vi "Scan Engine Custom IO - To FPGA.vi"(8 "error in (no error)":errorcluster, 11 "Node Ptr":T1 format="%.0x") -> (0 "error out":errorcluster)   [LabVIEW 2016, in "Scan Engine Custom Device.lvlib"]
uses:
  Scan Engine Custom Device.lvlib
  <vilib>/NI Veristand/Custom Device API/Custom Device Item Ref.ctl
  Type Defs/UDV Data Type.ctl
  Type Defs/FXP Config.ctl
  Globals/Property Strings.vi
  <vilib>/NI Veristand/Custom Device API/Get Item Property (String).vi
  <vilib>/NI Veristand/Custom Device API/Get Item Property (U16).vi
  <vilib>/NI Veristand/Custom Device API/Get Item Property (Variant).vi
  <vilib>/NI Veristand/Custom Device API/Custom Device API.lvlib
panel:
  out "IO Variable Name":string
  in  "Default Value":dbl
  in  "Units":string
  out "Data Type":string
  in  "Header":cluster{"Section Name":string}={"Section Name"="Custom FPGA I/O"}
  in  "Description":string
  in  "Name":string
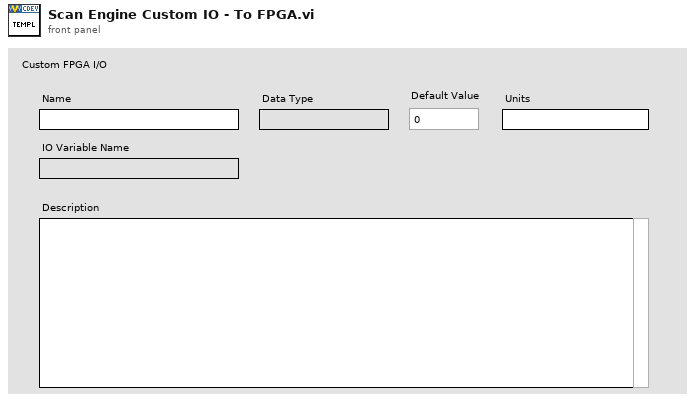
[diagram p1: front panel]
types:
  T1 = typedef "Custom Device API.lvlib/Custom Device Item Ref.ctl" = u64
  T2 = typedef "Scan Engine Custom Device.lvlib/UDV Data Type.ctl" = enum16{"Boolean", "Fixed Point", "Int8", "Int16", "Int32", "Int64", "U32 Bit Field", "UInt8", "UInt16", "UInt32", "UInt64", "Other"}
  T3 = typedef "Custom Device API.lvlib/Custom Device Item Info.ctl" = cluster{"Name":string, "Is Channel":bool, "GUID":string, "Is Waveform":bool}
  T4 = typedef "Custom Device API.lvlib/Custom Device Channel.ctl" = cluster{"Type":T5, "Units":string, "Default Value":dbl, "Faultable":bool, "Scalable":bool}
  T5 = typedef "Custom Device API.lvlib/Custom Device Channel Type.ctl" = enum16{"Input", "Output"}
  T6 = typedef "Scan Engine Custom Device.lvlib/FXP Config.ctl" = cluster{"signed":bool, "size":u32, "integersize":i32}
  T7 = typedef "Custom Device API.lvlib/Custom Device Commands.ctl" = enum16{"Default", "Item renamed", "Shutdown", "Dynamic button pressed"}
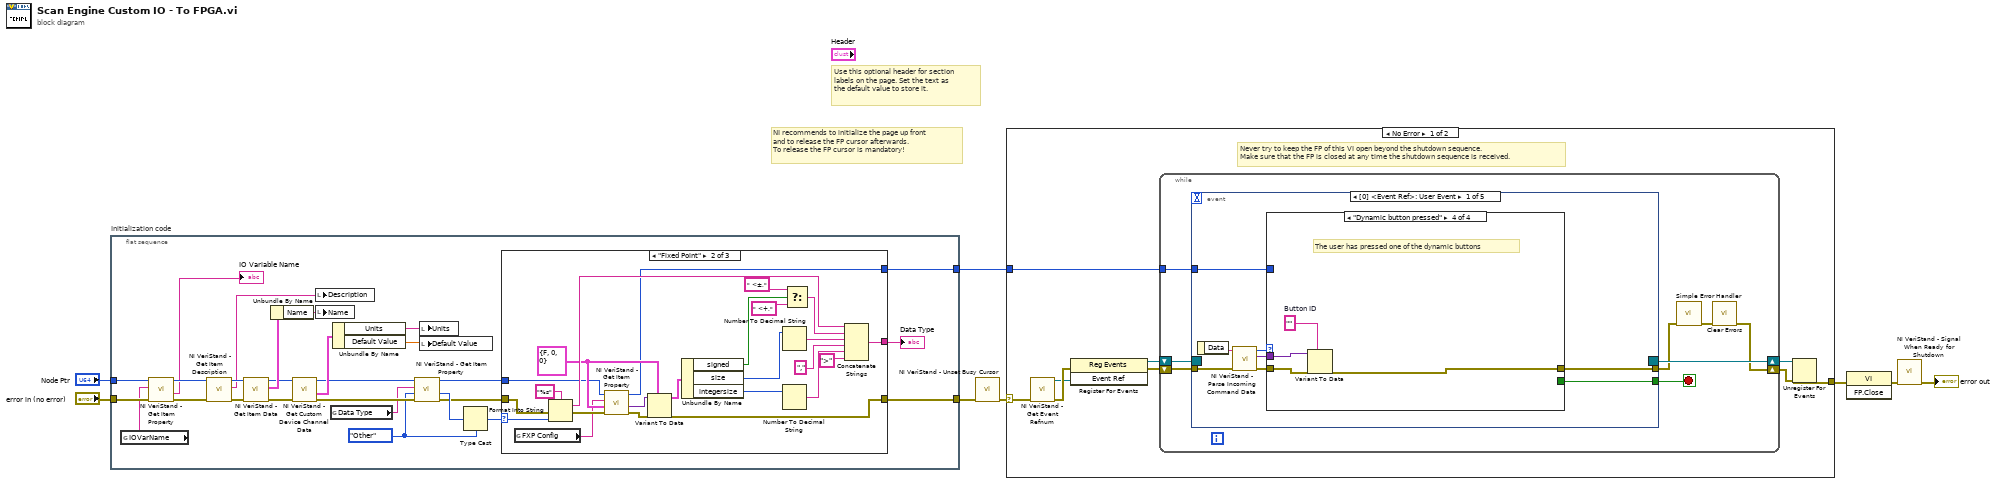
[diagram p0: block diagram]
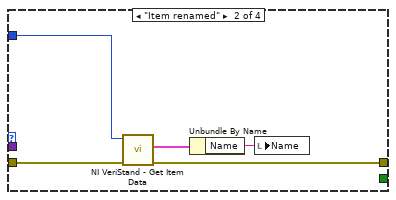
[diagram p3: hidden frame]
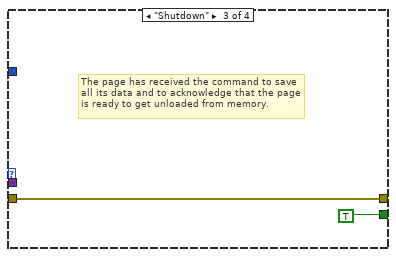
[diagram p4: hidden frame]
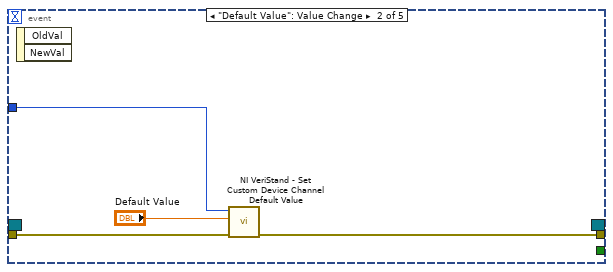
[diagram p5: hidden frame]
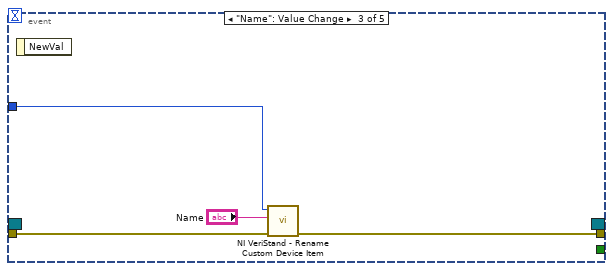
[diagram p6: hidden frame]
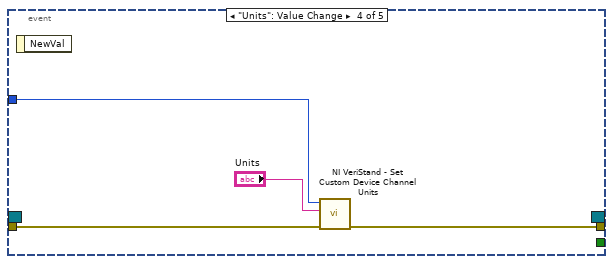
[diagram p7: hidden frame]
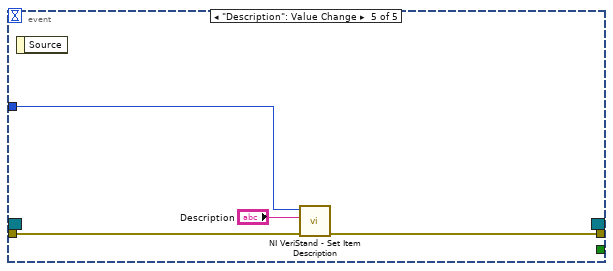
[diagram p8: hidden frame]
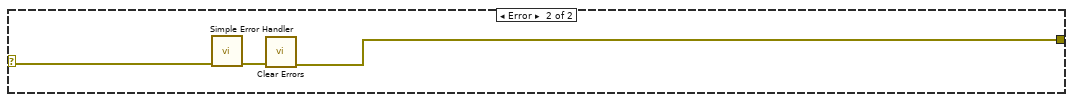
[diagram p9: hidden frame]
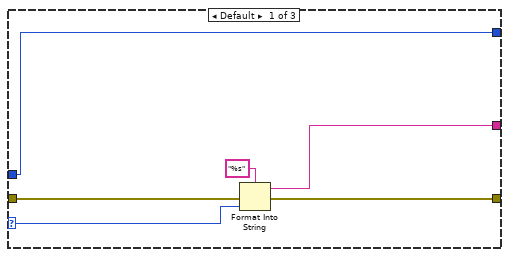
[diagram p10: hidden frame]
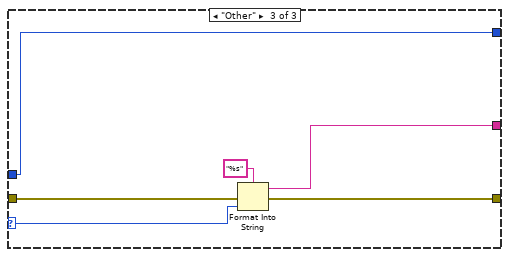
[diagram p11: hidden frame]
diagram:
  # "Use this optional header for section labels on the page. Set the text as the default value to store it."
  # "NI recommends to initialize the page up front\nand to release the FP cursor afterwards.\nTo release the FP cursor is mandatory!"
  n1 = flat-sequence "Initialization code" {
    tunnel: "error in (no error)" -> [w14]
    tunnel: "Node Ptr" -> [w12]
    tunnel: [w18] -> w4
    tunnel: [w16] -> w1
    frame #0 {
      w22 = UDV_Data_Type."Other" ("UDV Data Type out")
      n2 = global read "Property Strings.vi" "IOVarName"() -> (w9:string)
      n3 = call-poly <vilib>:"NI VeriStand - Get Item Property.vi"("error in (no error)"=w14, "Property Name"=w9, "Item Ref in"=w12) -> ("error out"=w13:errorcluster, "Value"=→"IO Variable Name":string, "Item Ref out"=w11:T1)  [unwired: 5 in, 1 out]
      n4 = call <vilib>:"NI VeriStand - Get Item Description.vi"("error in (no error)"=w13, "Item Ref in"=w11) -> ("error out"=w33:errorcluster, "Description"=w34:string, "Item Ref out"=w35:T1)  [unwired: 7 out]
      n5 = call <vilib>:"NI VeriStand - Get Item Data.vi"("error in (no error)"=w33, "Item Ref in"=w35) -> ("error out"=w29:errorcluster, "Item Info"=w32:T3, "Item Ref out"=w30:T1)  [unwired: 7 out]
      n6 = Unbundle By Name(w32) -> ("Name"=w31:string)
      n7 = call <vilib>:"NI VeriStand - Get Custom Device Channel Data.vi"("error in (no error)"=w29, "Channel Ref in"=w30) -> ("error out"=w25:errorcluster, "Channel"=w28:T4, "Channel Ref out"=w26:T1)  [unwired: 4 in, 3 out]
      n8 = local write "Description"(w34) -> ()
      n9 = local write "Name"(w31) -> ()
      n10 = global read "Property Strings.vi" "Data Type"() -> (w24:string)
      n11 = Unbundle By Name(w28) -> ("Units"=w27:string, "Default Value"=w15:dbl)
      n12 = call-poly <vilib>:"NI VeriStand - Get Item Property.vi"("error in (no error)"=w25, "Default Value"=w22, "Property Name"=w24, "Item Ref in"=w26) -> ("error out"=w21:errorcluster, "Value"=w23:u16, "Item Ref out"=w19:T1)  [unwired: 4 in, 1 out]
      n13 = local write "Units"(w27) -> ()
      n14 = local write "Default Value"(w15) -> ()
      n15 = Type Cast(type=w22, x=w23) -> (*(type *) &x=w20:T2)
      n16 = case shown="\"Fixed Point\"" w20 {
        selector: w20 -> [w40 w47 w69]
        tunnel: w21 -> [w41 w46 w70]
        tunnel: [w38 w43 w67] -> w17
        tunnel: [w37 w44 w68] -> w18
        tunnel: w19 -> [w36 w45 w66]
        tunnel: [w36 w42 w66] -> w16
        frame Default {
          n17 = Format Into String(format string="%s", error in=w41, w40) -> (resulting string=w38:string, error out=w37:errorcluster)  [unwired: 1 in]
        }
        frame "Fixed Point" {
          w51 = T6 {"signed"=FALSE, "size"=0, "integersize"=0} ("FXP Config")
          n18 = global read "Property Strings.vi" "FXP Config"() -> (w48:string)
          n19 = Format Into String(format string="%s", error in=w46, w47) -> (resulting string=w57:string, error out=w59:errorcluster)  [unwired: 1 in]
          n20 = call-poly <vilib>:"NI VeriStand - Get Item Property.vi"("error in (no error)"=w59, "Default Value"=w51, "Property Name"=w48, "Item Ref in"=w45) -> ("error out"=w49:errorcluster, "Value"=w50:variant, "Item Ref out"=w42:T1)  [unwired: 4 in, 1 out]
          n21 = Variant To Data(error in=w49, type=w51, Variant=w50) -> (data=w52:T6, error out=w44:errorcluster)
          n22 = Unbundle By Name(w52) -> ("signed"=w53:bool, "size"=w60:u32, "integersize"=w61:i32)
          n23 = Number To Decimal String(number=w60) -> (decimal integer string=w62:string)  [unwired: 1 in]
          n24 = Number To Decimal String(number=w61) -> (decimal integer string=w64:string)  [unwired: 1 in]
          n25 = Select(t=" <±,", s=w53, f=" <+,") -> (s? t:f=w58:string)
          n26 = Concatenate Strings(w57, w58, w62, ",", w64, ">") -> (w43:string)
        }
        frame "Other" {
          n27 = Format Into String(format string="%s", error in=w70, w69) -> (resulting string=w67:string, error out=w68:errorcluster)  [unwired: 1 in]
        }
      }
      "Data Type" <- w17
    }
  }
  n28 = call <vilib>:"NI VeriStand - Unset Busy Cursor.vi"("error in (no error)"=w4) -> ("error out"=w3:errorcluster)  [unwired: 10 out]
  n29 = case shown="No Error" w3 {
    selector: w3 -> [w73 w127]
    tunnel: [w77 w125] -> w8
    tunnel: w1 -> [w72 _]
    frame No Error {
      # "Never try to keep the FP of this VI open beyond the shutdown sequence.\nMake sure that the FP is closed at any time the shutdown sequence is received."
      n30 = call <vilib>:"NI VeriStand - Get Event Refnum.vi"("error in (no error)"=w73) -> ("error out"=w80:errorcluster, "Event Ref"=w76:refnum<user-event>)  [unwired: 9 out]
      n31 = register-events(error in=w80, w76) -> (reference out=w74:refnum<event-registration>, error out=w75:errorcluster)  [unwired: 1 in]
      n32 = while {
        shift-right: [w82] -> w78
        shift-left: w75 -> [w87]
        shift-right: [w88] -> w79
        shift-left: w74 -> [w86]
        tunnel: w72 -> [w81]
        stop <- w85 stop-if-true
        n33 = event shown="[0] <Event Ref>: User Event" {
          selector: w86 -> [_ _ _ _ _]
          dyn-events: [_ _ _ _ _] -> w88
          timeout: _ -> [_ _ _ _ _]
          tunnel: w87 -> [w96 w112 w116 w120 w124]
          tunnel: [w92 _ _ _ _] -> w85
          tunnel: [w91 w111 w115 w118 w123] -> w84
          tunnel: w81 -> [w89 w110 w113 w117 w121]
          event User Event {
            n34 = event-data() -> ("Data"=w95:string)  [unwired: 1 out]
            n35 = call <vilib>:"NI VeriStand - Parse Incoming Command Data.vi"("error in (no error)"=w96, "Incoming data"=w95) -> ("error out"=w94:errorcluster, "Outgoing data"=w90:variant, "Action"=w93:T7)  [unwired: 7 out]
            n36 = case shown="\"Dynamic button pressed\"" w93 {
              tunnel: w94 -> [w97 w102 w103 w108]
              tunnel: [_ _ TRUE _] -> w92
              tunnel: [w97 w100 w103 w105] -> w91
              tunnel: w90 -> [_ _ _ w107]
              tunnel: w89 -> [_ w98 _ _]
              frame "Default", Default {
              }
              frame "Item renamed" {
                n37 = call <vilib>:"NI VeriStand - Get Item Data.vi"("error in (no error)"=w102, "Item Ref in"=w98) -> ("error out"=w100:errorcluster, "Item Info"=w101:T3)  [unwired: 8 out]
                n38 = Unbundle By Name(w101) -> ("Name"=w99:string)
                n39 = local write "Name"(w99) -> ()
              }
              frame "Shutdown" {
                # "The page has received the command to save all its data and to acknowledge that the page is ready to get unloaded from memory."
              }
              frame "Dynamic button pressed" {
                w106 = ""  # Button ID
                # "The user has pressed one of the dynamic buttons"
                n40 = Variant To Data(error in=w108, type=w106, Variant=w107) -> (error out=w105:errorcluster)  [unwired: 1 out]
              }
            }
          }
          event "Default Value": Value Change {
            n41 = event-data() -> ()  [unwired: 3 out]
            n42 = call <vilib>:"NI VeriStand - Set Custom Device Channel Default Value.vi"("error in (no error)"=w112, "Default Value"="Default Value", "Channel Ref in"=w110) -> ("error out"=w111:errorcluster)  [unwired: 7 in, 1 out]
          }
          event "Name": Value Change {
            n43 = event-data() -> ()  [unwired: 2 out]
            n44 = call <vilib>:"NI VeriStand - Rename Custom Device Item.vi"("error in (no error)"=w116, "New Name"="Name", "Item Ref in"=w113) -> ("error out"=w115:errorcluster)  [unwired: 1 in, 7 out]
          }
          event "Units": Value Change {
            n45 = event-data() -> ()  [unwired: 2 out]
            n46 = call <vilib>:"NI VeriStand - Set Custom Device Channel Units.vi"("error in (no error)"=w120, "Units"="Units", "Channel Ref in"=w117) -> ("error out"=w118:errorcluster)  [unwired: 7 in, 1 out]
          }
          event "Description": Value Change {
            n47 = event-data() -> ()  [unwired: 2 out]
            n48 = call <vilib>:"NI VeriStand - Set Item Description.vi"("error in (no error)"=w124, "Description"="Description", "Item Ref in"=w121) -> ("error out"=w123:errorcluster)  [unwired: 8 out]
          }
        }
        n49 = call <vilib>:"Simple Error Handler.vi"("error in (no error)"=w84) -> ("error out"=w83:errorcluster)  [unwired: 1 in, 7 out]
        n50 = call <vilib>:"Clear Errors.vi"("error in (no error)"=w83) -> ("error out"=w82:errorcluster)  [unwired: 1 in, 5 out]
      }
      n51 = Unregister For Events(event registration refnum=w79, error in=w78) -> (error out=w77:errorcluster)
    }
    frame Error {
      n52 = call <vilib>:"Simple Error Handler.vi"("error in (no error)"=w127) -> ("error out"=w126:errorcluster)  [unwired: 1 in, 7 out]
      n53 = call <vilib>:"Clear Errors.vi"("error in (no error)"=w126) -> ("error out"=w125:errorcluster)  [unwired: 1 in, 5 out]
    }
  }
  n54 = invoke class="VI" method="FP.Close"(error in=w8) -> (error out=w7:errorcluster)  [unwired: 2 in, 2 out]
  n55 = call <vilib>:"NI VeriStand - Signal When Ready for Shutdown.vi"("error in (no error)"=w7) -> ("error out"=→"error out":errorcluster)  [unwired: 10 out]
